vi "GeneradorConboton.vi"() -> ()   [LabVIEW 2021]
panel:
  out "Waveform Chart":dbl(graph)
  in  "Knob":dbl(knob) scale=0.1..2.0
  in  "Boolean":bool
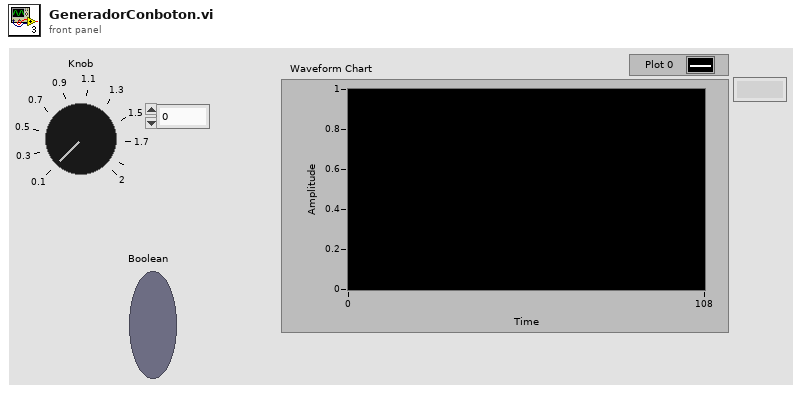
[diagram p1: front panel]
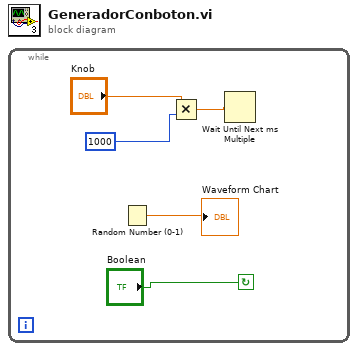
[diagram p0: block diagram]
diagram:
  n1 = while {
    stop <- "Boolean" continue-if-true
    n2 = Random Number (0-1)() -> (number: 0 to 1=→"Waveform Chart":dbl)
    n3 = Multiply(x="Knob", y=1000) -> (x*y=w4:dbl)
    n4 = Wait Until Next ms Multiple(millisecond multiple=w4) -> ()  [unwired: 1 out]
  }
